vi "Set Setpoint Slope--SubVI.vi"(8 "error in (no error)":errorcluster, 9 "Setpoint Slope":u16, 10 "Device":T9, 11 "Data Cluster":T1 {"Flexi-Flow Devices"."Control State"."Control Mode" items=["Bus/RS232"=0, "FLOW-BUS slave"=2, "Valve close"=3, "Controller idle"=4, "Setpoint 100%"=7, "Valve fully open"=8, "Calibration mode"=9, "Setpoint 0%"=12, "RS232"=18, "Valve steering"=20, "Valve safe state"=22]}) -> (0 "error out":errorcluster, 3 "Data Cluster Out":T1 {"Flexi-Flow Devices"."Control State"."Control Mode" items=["Bus/RS232"=0, "FLOW-BUS slave"=2, "Valve close"=3, "Controller idle"=4, "Setpoint 100%"=7, "Valve fully open"=8, "Calibration mode"=9, "Setpoint 0%"=12, "RS232"=18, "Valve steering"=20, "Valve safe state"=22]})   [LabVIEW 2024, in "FlexiFlowInterface.lvlib"]
uses:
  FlexiFlowInterface.lvlib
  Module Data--cluster.ctl
  Modbus TCP Connection Settings--cluster.ctl
  Modbus Flexi-Flow State--cluster.ctl
  <vilib>/Plasmionique/MB Master/MB_Master_TCP/MB_Master_TCP.lvclass
  Device Type--enum.ctl
  Modbus Flexi-Flow Controls--cluster.ctl
  Modbus Flexi-Flow API/Control Mode--enum.ctl
  Modbus Flexi-Flow API/Control Function Values--enum.ctl
  Modbus Flexi-Flow Measure State--cluster.ctl
  FlexiFlowDevice--enum.ctl
  Modbus Flexi-Flow API/PDU Address U16 Params--ring.ctl
  Modbus Flexi-Flow API/Write Unsigned Int Register.vi
  Modbus Flexi-Flow API/Read Unsigned Int Register.vi
  Modbus Flexi-Flow API/Bronkhorst Flexi-Flow ModbusTCP API.lvlib
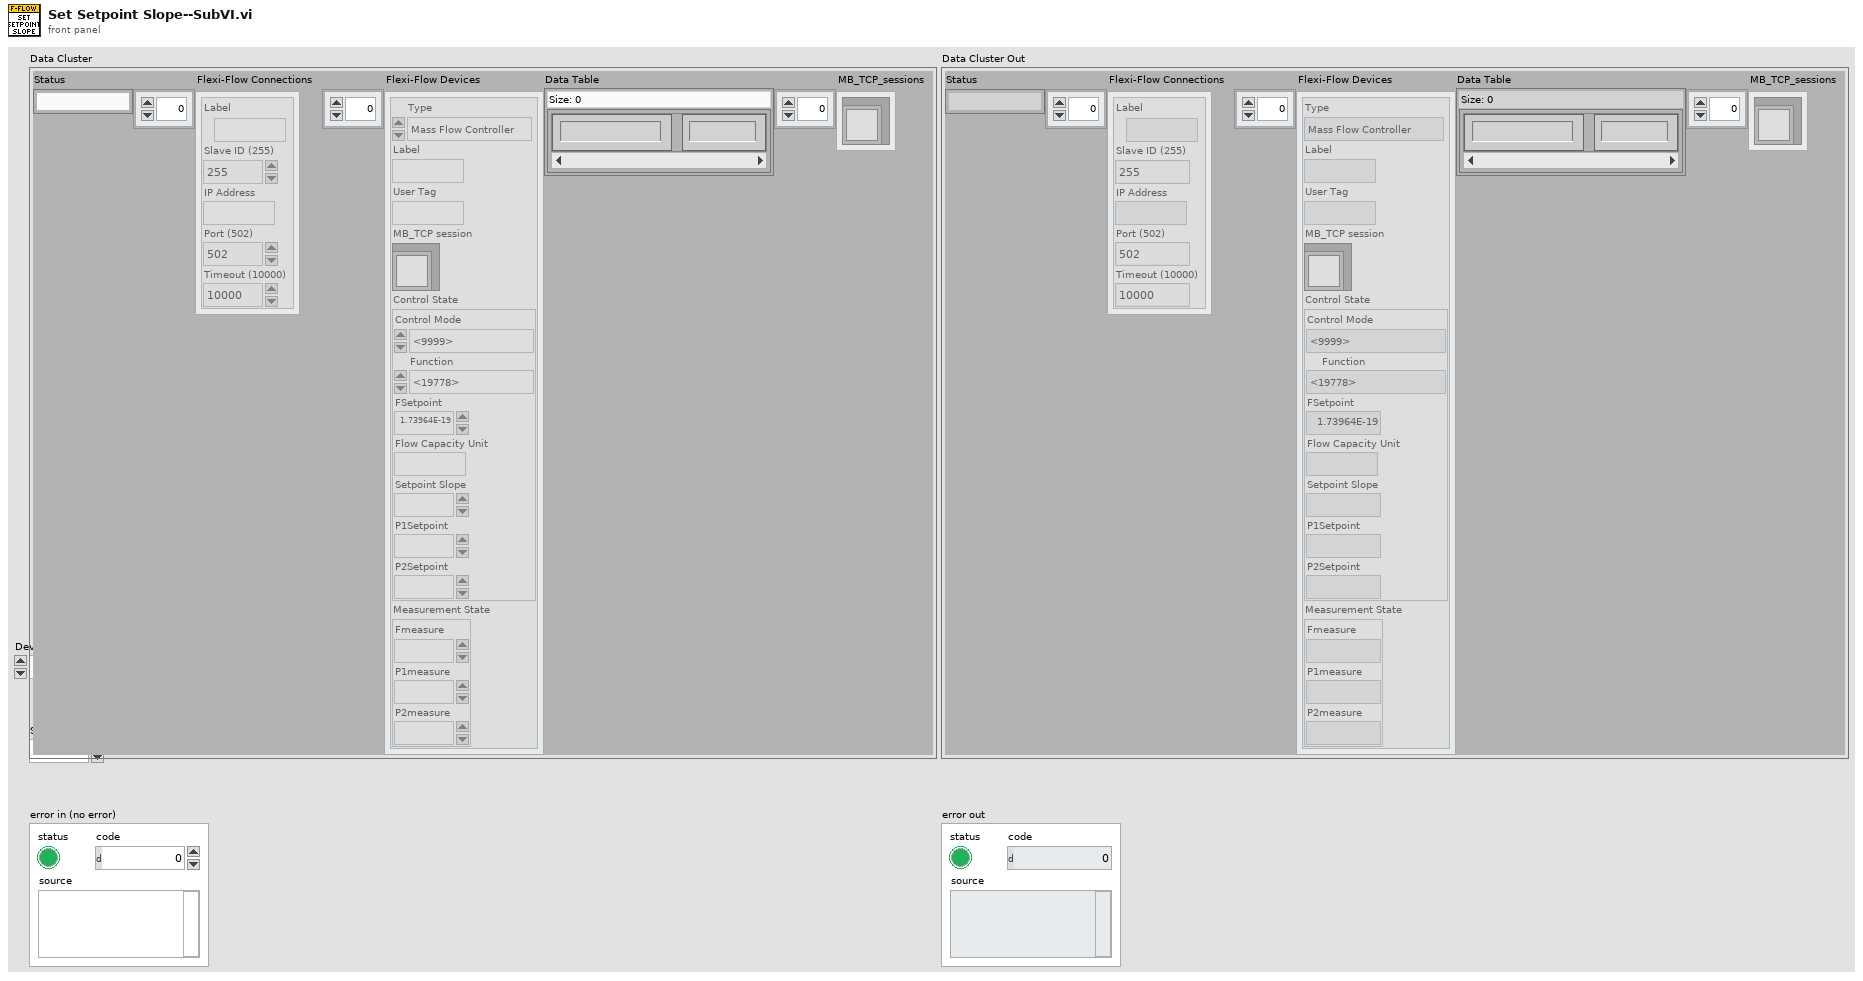
[diagram p1: front panel]
types:
  T1 = typedef "FlexiFlowInterface.lvlib/Module Data--cluster.ctl" = cluster{"Status":string, "Flexi-Flow Connections":T2[], "Flexi-Flow Devices":T3[], "Data Table":map{string, dbl}, "MB_TCP_sessions":refnum<class "MB_Master_TCP.lvclass">[]}
  T2 = typedef "FlexiFlowInterface.lvlib/Modbus TCP Connection Settings--cluster.ctl" = cluster{"Label":string, "Slave ID (255)":u8, "IP Address":string, "Port (502)":u16, "Timeout (10000)":i32}
  T3 = typedef "FlexiFlowInterface.lvlib/Modbus Flexi-Flow State--cluster.ctl" = cluster{"Type":T4, "Label":string, "User Tag":string, "MB_TCP session":refnum<class "MB_Master_TCP.lvclass">, "Control State":T5, "Measurement State":T8}
  T4 = typedef "FlexiFlowInterface.lvlib/Device Type--enum.ctl" = enum16{"Mass Flow Controller", "Mass Flow Meter"}
  T5 = typedef "FlexiFlowInterface.lvlib/Modbus Flexi-Flow Controls--cluster.ctl" = cluster{"Control Mode":T6, "Function":T7, "FSetpoint":sgl, "Flow Capacity Unit":string, "Setpoint Slope":u16, "P1Setpoint":sgl, "P2Setpoint":sgl}
  T6 = typedef "Bronkhorst Flexi-Flow ModbusTCP API.lvlib/Control Mode--enum.ctl" = u16
  T7 = typedef "Bronkhorst Flexi-Flow ModbusTCP API.lvlib/Control Function Values--enum.ctl" = enum16{"Flow", "Upstream pressure", "Downstream pressure", "Flow with upstream pressure limit", "Flow with downstream pressure limit", "Upstream pressure with flow limit", "Downstream pressure with flow limit"}
  T8 = typedef "FlexiFlowInterface.lvlib/Modbus Flexi-Flow Measure State--cluster.ctl" = cluster{"Fmeasure":dbl, "P1measure":sgl, "P2measure":sgl}
  T9 = typedef "FlexiFlowInterface.lvlib/FlexiFlowDevice--enum.ctl" = enum16{"Hydrogen Inlet", "Nitrogen Inlet", "Cathode Outlet", "Anode Outlet"}
  T10 = typedef "Bronkhorst Flexi-Flow ModbusTCP API.lvlib/PDU Address U16 Params--ring.ctl" = u16
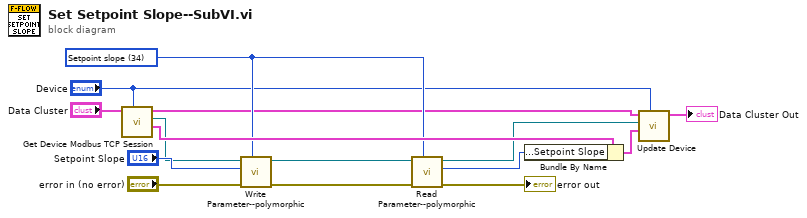
[diagram p0: block diagram]
diagram:
  w11 = T10 34 items=["Setpoint"=33, "Setpoint slope"=34, "Alarm limit maximum"=3105, "Alarm limit minimum"=3106, "Alarm new setpoint"=3110, "Counter limit (UInt)"=3331, "Counter new setpoint"=3334, "Valve output"=61960, "Control Function"=3690, "TEMP"=0] ("PDU Address (U-Int16)")
  n1 = call "Get Device Modbus TCP Session.vi"("Device"="Device", "Data Cluster In"="Data Cluster") -> ("Device State"=w13:T3, "MB_TCP session"=w6:refnum<class "MB_Master_TCP.lvclass">, "Data Cluster Out"=w1:T1)  [unwired: 7 in]
  n2 = call-poly "Write Parameter--polymorphic.vi"("PDU Address (U-Int16)"=w11, "error in"="error in (no error)", "Value"="Setpoint Slope", "MB_TCP session in"=w6) -> ("error out"=w4:errorcluster, "MB session out"=w10:refnum<class "MB_Master_TCP.lvclass">)  [unwired: 6 in]
  n3 = call-poly "Read Parameter--polymorphic.vi"("PDU Address (U-Int16)"=w11, "error in"=w4, "MB_TCP session in"=w10) -> ("error out"=→"error out":errorcluster, "Value"=w15:u16, "MB session out"=w9:refnum<class "MB_Master_TCP.lvclass">)  [unwired: 6 in]
  n4 = Bundle By Name(cluster=w13, "Control State.Setpoint Slope"=w15) -> (w14:T3)
  n5 = call "Update Device.vi"("Device"="Device", "Device State"=w14, "MB_TCP session"=w9, "Data Cluster"=w1) -> ("Data Cluster Out"=→"Data Cluster Out":T1)  [unwired: 7 in]
